vi "2DLIF.Colors.vi"(6 "override scale?":bool=TRUE, 7 "Intensity Graph":i32[][](array[numeric]), 9 "manual max":i32=50000, 10 "manual min":i32=24200, 11 "ZScale.Range in":T1) -> (1 "min/max":i32[](array[numeric])=[153385, 23581], 2 "Zscale.MarkerVals[]":cluster{dbl, u32}[](array[cluster]), 3 "ZScale.Range out":T1)   [LabVIEW 2022 SP3]
uses:
  <vilib>/Utility/miscctls.llb/LVRangeTypeDef.ctl
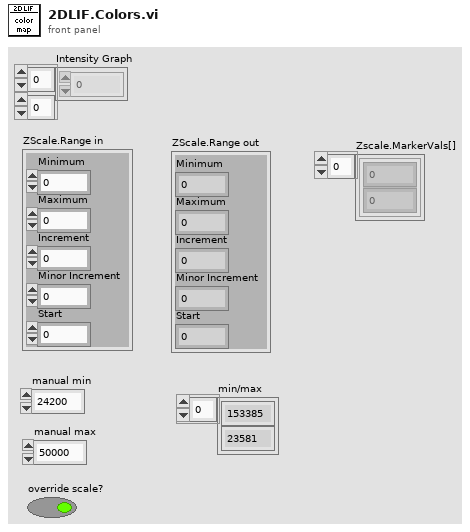
[diagram p1: front panel]
types:
  T1 = typedef "LVRangeTypeDef.ctl" = cluster{"Minimum":dbl, "Maximum":dbl, "Increment":dbl, "Minor Increment":dbl, "Start":dbl}
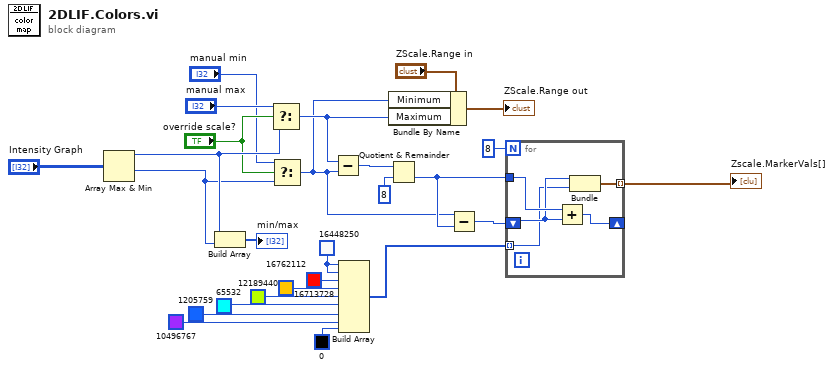
[diagram p0: block diagram]
diagram:
  w20 = u32 16448250
  n1 = Array Max & Min(array="Intensity Graph") -> (max value=w10:i32, min value=w7:i32)  [unwired: 2 out]
  n2 = Build Array(w10, w7) -> (→"min/max":i32[])
  n3 = Select(t="manual max", s="override scale?", f=w10) -> (s? t:f=w8:i32)
  n4 = Select(t="manual min", s="override scale?", f=w7) -> (s? t:f=w1:i32)
  n5 = Subtract(x=w8, y=w1) -> (x-y=w4:i32)
  n6 = Build Array(w20, w20, u32 16713728, u32 16762112, u32 12189440, u32 65532, u32 1205759, u32 10496767, u32 0) -> (w15:u32[])
  n7 = Bundle By Name(cluster="ZScale.Range in", "Minimum"=w1, "Maximum"=w8) -> (→"ZScale.Range out":T1)
  n8 = Quotient & Remainder(x=w4, y=8) -> (floor(x/y)=w2:i32)  [unwired: 1 out]
  n9 = Subtract(x=w1, y=w2) -> (x-y=w23:i32)
  n10 = for {
    N: 8 -> [_]
    shift-right: [w27] -> _
    shift-left: w23 -> [w30]
    tunnel: w2 -> [w31]
    tunnel: w15 -> [w29] mode=indexing
    tunnel: [w28] -> w14 mode=indexing
    n11 = Add(x=w31, y=w30) -> (x+y=w27:i32)
    n12 = Bundle(w30, w29) -> (w28:cluster{i32, u32})  [unwired: 1 in]
  }
  "Zscale.MarkerVals[]" <- w14
